vi "SwitchedACIR.vi"(5 "Switch":refnum<class "Switch.lvclass">, 6 "Setting":T1={"Freq"=1000.0, "Range"=enum."10m Ohm", "Measurements"=enum."OCV"} {"Freq" min=0.1 max=1050.0 step=0.01 format="%_5e"}, 7 "Analog In":refnum<class "Analog In.lvclass">, 8 "error in":errorcluster, 9 "Connection(s)":string="102", 10 "Switch Ref":string, 11 "ACIR Ref":string) -> (0 "error out":errorcluster, 1 "Measurements":dbl[](array[numeric]), 2 "Switch out":refnum<class "Switch.lvclass">, 3 "Analog In out":refnum<class "Analog In.lvclass">)   [LabVIEW 2019, in "Code Modules.lvlib"]
uses:
  Code Modules.lvlib
  PPLs/Hardware Abstraction.lvlibp/Harware Abstraction/Switch/Switch.lvclass
  PPLs/Hardware Abstraction.lvlibp/Harware Abstraction/Analog In/Analog In.lvclass
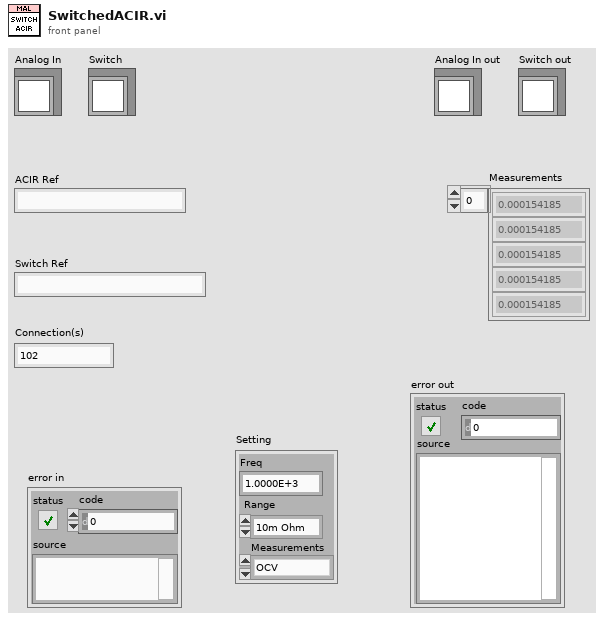
[diagram p1: front panel]
types:
  T1 = cluster{"Freq":dbl, "Range":enum16{"3m Ohm", "10m Ohm", "100m Ohm"}, "Measurements":enum16{"Impedence", "Phase Angle", "OCV"}}
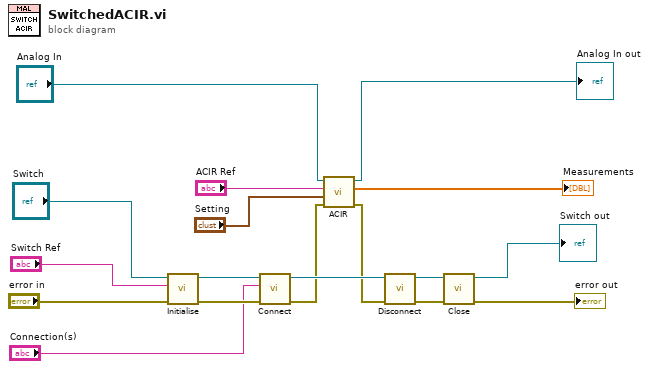
[diagram p0: block diagram]
diagram:
  n1 = call-dynamic "Initialise.vi"("error in (no error)"="error in", "Instrument Ref"="Switch Ref", "Instrument in"="Switch") -> ("error out"=w9:errorcluster, "Instrument out"=w11:refnum<class "Switch.lvclass">)  [unwired: 7 in]
  n2 = call-dynamic "Connect.vi"("error in (no error)"=w9, "Channel(s)"="Connection(s)", "Switch in"=w11) -> ("error out"=w2:errorcluster, "Switch out"=w12:refnum<class "Switch.lvclass">)  [unwired: 7 in]
  n3 = call "ACIR.vi"("error in"=w2, "Setting"="Setting", "ACIR Ref"="ACIR Ref", "Analog In"="Analog In") -> ("error out"=w1:errorcluster, "Measurements"=→"Measurements":dbl[], "Analog In"=→"Analog In out":refnum<class "Analog In.lvclass">)  [unwired: 5 in]
  n4 = call-dynamic "Disconnect.vi"("error in (no error)"=w1, "Switch in"=w12) -> ("error out"=w10:errorcluster, "Switch out"=w13:refnum<class "Switch.lvclass">)  [unwired: 8 in]
  n5 = call-dynamic "Close.vi"("error in (no error)"=w10, "Instrument in"=w13) -> ("error out"=→"error out":errorcluster, "Instrument out"=→"Switch out":refnum<class "Switch.lvclass">)  [unwired: 8 in]
